vi "3_MathTest.vi"() -> ()   [LabVIEW 2012]
panel:
  out "BotSpeak":string="SET count1,1\nADD count1,1\nADD count1,count1\nSCRIPT\nSET tmp0,4\nDIV tmp0,2\nSET paren1,3\nADD paren1,tmp0\nSET paren0,5\nSUB paren0,3\nSET tmp1,2\nMUL tmp1,paren0\nSET tmp2,5\nMUL tmp2,paren1\nSET sum,tmp1\nSET tmp3,1\nSUB tmp3,tmp2\nADD sum,tmp3\nSET tmp0,2\nBSL tmp0,2\nSET more,5\nMOD more,tmp0\nSET X,6\nDIV X,2\nend\nENDSCRIPT\nRUN&WAIT 0\nGET sum\nGET more\nGET X\n\n"
  out "expected response":string="1\r\n2\r\n4\r\nstart script\r\nend script\r\n.....................\nDone\r\n-20\r\n5\r\n3\r\n"
  out "response":string="1\r\n2\r\n4\r\nstart script\r\nend script\r\n.....................\nDone\r\n-20\r\n5\r\n3\r\n"
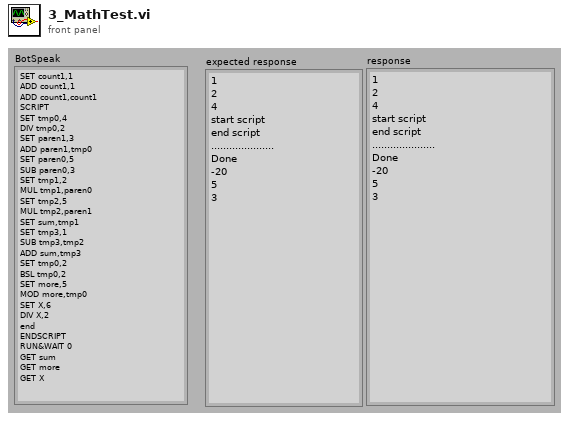
[diagram p1: front panel]
types:
  T1 = typedef "BotSpeak_Control.ctl" = cluster{"Address":string, "Reply EOF":string, "Hardware":path, "Retries":i8, "Timeout":i32}
  T2 = typedef "URAPI_Control.ctl" = cluster{"Script":string, "Whiles":u8[], "Ifs":u8[], "Supress Err":bool, "Errors":string}
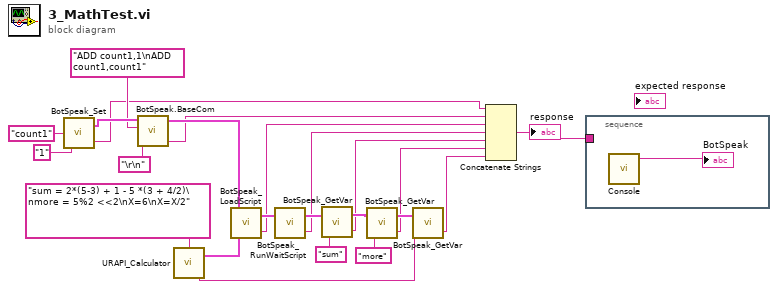
[diagram p0: block diagram]
diagram:
  n1 = call <userlib>:"BotSpeak_Set.vi"("value"="1", "Variable In"="count1") -> ("response"=w8:string, "Bot Settings"=w20:T1)  [unwired: 1 in]
  n2 = call <userlib>:"BotSpeak.BaseCom.vi"("Termination"="\r\n", "command"="ADD count1,1\nADD count1,count1" ("String"), "Bot Settings in"=w20) -> ("response"=w7:string, "Bot Settings out"=w16:T1)  [unwired: 2 in]
  n3 = call <userlib>:"URAPI_Calculator.vi"("Formula"="sum = 2*(5-3) + 1 - 5 *(3 + 4/2)\nmore = 5%2 <<2\nX=6\nX=X/2") -> ("Variable Out"=w9:string, "URAPI Script"=w17:T2)  [unwired: 3 in]
  n4 = call <userlib>:"BotSpeak_LoadScript.vi"("URAPI Script"=w17, "Bot Settings"=w16) -> ("total response"=w6:string, "Bot Settings"=w15:T1)
  n5 = call <userlib>:"BotSpeak_RunWaitScript.vi"("Bot Settings"=w15) -> ("response"=w5:string, "Bot Settings"=w14:T1)  [unwired: 1 in]
  n6 = call <userlib>:"BotSpeak_GetVar.vi"("Variable In"="sum", "Bot Settings"=w14) -> ("value"=w4:string, "Bot Settings out"=w11:T1)
  n7 = call <userlib>:"BotSpeak_GetVar.vi"("Variable In"="more", "Bot Settings"=w11) -> ("value"=w3:string, "Bot Settings out"=w10:T1)
  n8 = call <userlib>:"BotSpeak_GetVar.vi"("Variable In"=w9, "Bot Settings"=w10) -> ("value"=w2:string)  [unwired: 1 out]
  n9 = Concatenate Strings(w8, w7, w6, w5, w4, w3, w2) -> (w1:string)
  "response" <- w1
  n10 = stacked-sequence {
    tunnel: w1 -> [_]
    frame #0 {
      n11 = call <userlib>:"Console.vi"() -> ("BotSpeak"=→"BotSpeak":string)  [unwired: 4 in, 1 out]
    }
  }
